vi "SMO.UI.Example.TestLauncher.vi"() -> ()   [LabVIEW 2013, in "SMO.UI.Example.lvclass"]
uses:
  SMO.UI.Example.lvclass
  src/SMO/SMO.lvclass
  src/SMO.UI/SMO.UI.lvclass
panel:
  out "error out":errorcluster
  in  "Stop":bool
  # "SMO.UI Test Launcher"
  # "For instructions on how to use the JKI State Machine Objects, examples and video tutorials, visit:\nhttp://jki.net/state-machine-objects/\n\nJKI State Machine Objects™\nhttp://jki.net/state-machine-objects/\nCopyright (C) 2005-2015, JKI <info@jki.net>\nALL RIGHTS RESERVED"
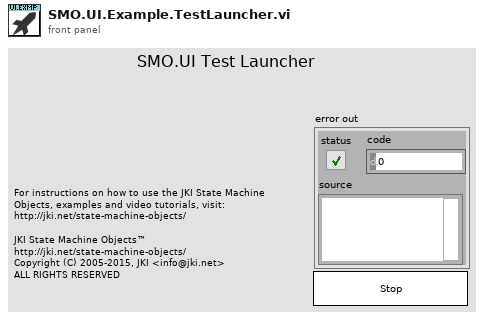
[diagram p1: front panel]
types:
  T1 = cluster{"SMO.UI Public Events":refnum<event-registration>}
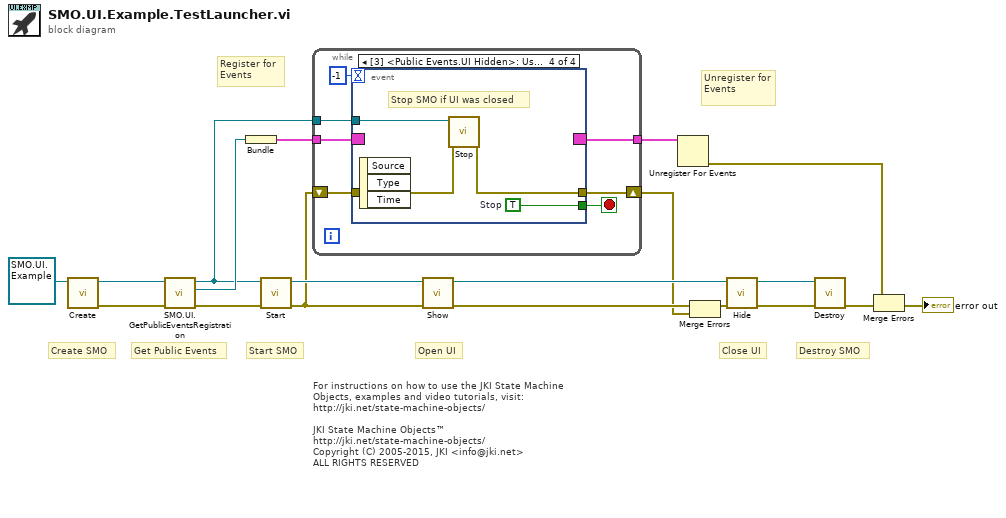
[diagram p0: block diagram]
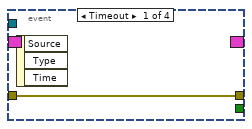
[diagram p2: hidden frame]
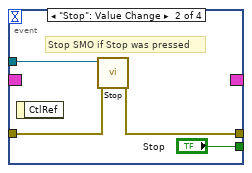
[diagram p3: hidden frame]
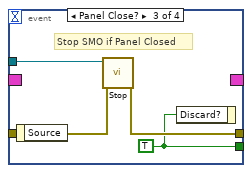
[diagram p4: hidden frame]
diagram:
  # "For instructions on how to use the JKI State Machine Objects, examples and video tutorials, visit:\nhttp://jki.net/state-machine-objects/\n\nJKI State Machine Objects™\nhttp://jki.net/state-machine-objects/\nCopyright (C) 2005-2015, JKI <info@jki.net>\nALL RIGHTS RESERVED"
  # "Get Public Events"
  # "Start SMO"
  # "Destroy SMO"
  # "Create SMO"
  # "Close UI"
  # "Open UI"
  # "Unregister for Events"
  # "Register for Events"
  n1 = call "Create.vi"("SMO"=refnum<class "SMO.UI.Example.lvclass"> refnum ("SMO.UI.Example.lvclass")) -> ("error out"=w2:errorcluster, "SMO out"=w1:refnum<class "SMO.UI.Example.lvclass">)  [unwired: 8 in, 1 out]
  n2 = call "SMO.UI.GetPublicEventsRegistration.vi"("error in (no error)"=w2, "SMO.UI"=w1) -> ("error out"=w18:errorcluster, "SMO.UI Public Events"=w17:refnum<event-registration>, "SMO.UI out"=w9:refnum<class "SMO.UI.Example.lvclass">)  [unwired: 7 in]
  n3 = Bundle("SMO.UI Public Events"=w17) -> (w16:T1)  [unwired: 1 in]
  n4 = call "Start.vi"("error in (no error)"=w18, "SMO"=w9) -> ("error out"=w11:errorcluster, "SMO out"=w15:refnum<class "SMO.UI.Example.lvclass">)  [unwired: 8 in]
  n5 = while {
    shift-right: [w25] -> w10
    shift-left: w11 -> [w24]
    tunnel: w16 -> [w23]
    tunnel: [w22] -> w19
    tunnel: w9 -> [w21]
    stop <- w26 stop-if-true
    n6 = event shown="[3] <Public Events.UI Hidden>: User Event" {
      selector: w23 -> [_ _ _ _]
      dyn-events: [_ _ _ _] -> w22
      timeout: -1 -> [_ _ _ _]
      tunnel: [_ "Stop" w32 w36] -> w26
      tunnel: w21 -> [_ w29 w35 w39]
      tunnel: [w27 w30 w34 w38] -> w25
      tunnel: w24 -> [w27 w28 w33 w37]
      event Timeout {
        n7 = event-data() -> ()  [unwired: 1 in, 3 out]
      }
      event "Stop": Value Change {
        # "Stop SMO if Stop was pressed"
        n8 = event-data() -> ()  [unwired: 1 in, 1 out]
        n9 = call "Stop.vi"("error in (no error)"=w28, "SMO"=w29) -> ("error out"=w30:errorcluster)  [unwired: 8 in, 1 out]
      }
      event Panel Close? {
        w32 = TRUE ("OK")
        # "Stop SMO if Panel Closed"
        n10 = event-data() -> ()  [unwired: 1 in, 1 out]
        n11 = call "Stop.vi"("error in (no error)"=w33, "SMO"=w35) -> ("error out"=w34:errorcluster)  [unwired: 8 in, 1 out]
        n12 = event-data("Discard?"=w32) -> ()  [unwired: 1 in, 1 out]
      }
      event User Event {
        w36 = TRUE  # Stop
        # "Stop SMO if UI was closed"
        n13 = event-data() -> ()  [unwired: 1 in, 3 out]
        n14 = call "Stop.vi"("error in (no error)"=w37, "SMO"=w39) -> ("error out"=w38:errorcluster)  [unwired: 8 in, 1 out]
      }
    }
  }
  n15 = call "Show.vi"("error in (no error)"=w11, "SMO.UI"=w15) -> ("error out"=w14:errorcluster, "SMO.UI out"=w13:refnum<class "SMO.UI.Example.lvclass">)  [unwired: 8 in]
  n16 = Unregister For Events(event registration refnum=w19) -> (error out=w8:errorcluster)  [unwired: 1 in]
  n17 = Merge Errors(w14, w10) -> (w12:errorcluster)
  n18 = call "Hide.vi"("error in (no error)"=w12, "SMO.UI"=w13) -> ("error out"=w5:errorcluster, "SMO.UI out"=w4:refnum<class "SMO.UI.Example.lvclass">)  [unwired: 8 in]
  n19 = call "Destroy.vi"("error in (no error)"=w5, "SMO"=w4) -> ("error out"=w3:errorcluster)  [unwired: 9 in]
  n20 = Merge Errors(w8, w3) -> (→"error out":errorcluster)
